vi "Deserialize.vi"(8 "error in (no error)":errorcluster, 10 "CI Deserializer in":refnum<class "CI Deserializer.lvclass">) -> (0 "error out":errorcluster, 2 "CI Deserializer out":refnum<class "CI Deserializer.lvclass">, 3 "Node out":T1)   [LabVIEW 2014, in "CI Deserializer.lvclass"]
uses:
  CI Deserializer.lvclass
  <vilib>/ni/Configuration Framework/Node/NodeRef.ctl
  <vilib>/ni/Configuration Framework/Node/NISE_CEF_Node.lvclass
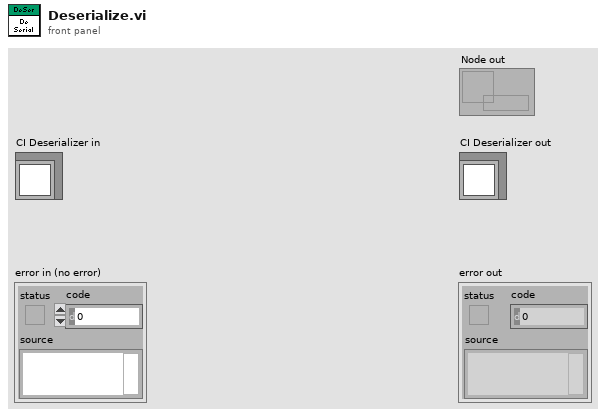
[diagram p1: front panel]
types:
  T1 = typedef "NISE_CEF_Node.lvclass/NodeRef.ctl" = refnum<data-value>
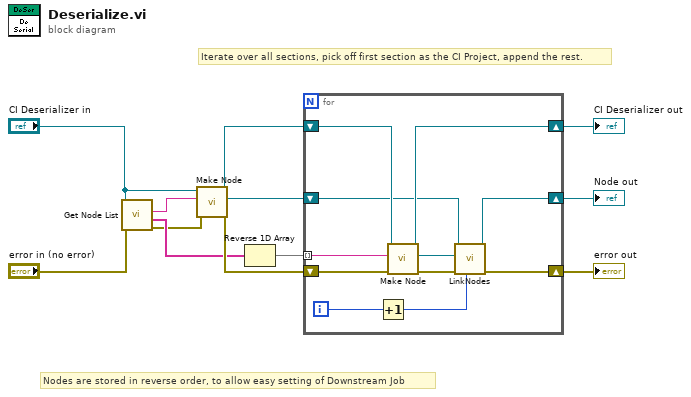
[diagram p0: block diagram]
diagram:
  # "Nodes are stored in reverse order, to allow easy setting of Downstream Job"
  # "Iterate over all sections, pick off first section as the CI Project, append the rest."
  n1 = call-dynamic "Get Node List.vi"("error in (no error)"="error in (no error)", "CI Deserializer in"="CI Deserializer in") -> ("error out"=w1:errorcluster, "Subnodes"=w5:string[], "Root Node"=w4:string)  [unwired: 7 in]
  n2 = call "Make Node.vi"("error in (no error)"=w1, "Node Name"=w4, "CI Deserializer in"="CI Deserializer in") -> ("error out"=w10:errorcluster, "Node Reference"=w12:refnum<data-value>, "CI Deserializer out"=w11:refnum<class "CI Deserializer.lvclass">)  [unwired: 6 in]
  n3 = Reverse 1D Array(array=w5) -> (reversed array=w2:string[])
  n4 = for {
    shift-right: [w20] -> w9
    shift-left: w11 -> [w21]
    tunnel: w2 -> [w22] mode=indexing
    shift-right: [w16] -> w7
    shift-left: w10 -> [w23]
    shift-right: [w15] -> w8
    shift-left: w12 -> [w18]
    i -> [w14]
    n5 = Increment(x=w14) -> (x+1=w13:i32)
    n6 = call "Make Node.vi"("error in (no error)"=w23, "Node Name"=w22, "CI Deserializer in"=w21) -> ("error out"=w19:errorcluster, "Node Reference"=w17:refnum<data-value>, "CI Deserializer out"=w20:refnum<class "CI Deserializer.lvclass">)  [unwired: 6 in]
    n7 = call <vilib>:"LinkNodes.vi"("index"=w13, "error in"=w19, "child in"=w17, "parent in"=w18) -> ("error out"=w16:errorcluster, "parent out"=w15:T1)  [unwired: 5 in, 1 out]
  }
  "error out" <- w7
  "CI Deserializer out" <- w9
  "Node out" <- w8
